vi "Perform measurements.vi"(6 "measurement configuration":T3={"Input channel"=0, "Full scale range"=10.0, "Analog source resource name"="", "Frequency"=1000.0, "Amplitude"=-1.0, "Digital capture resource name"="", "Digital capture sample rate"=800000.0, "Digital capture samples"=800000}, 11 "gRPC ID Out":T1) -> (0 "error out":errorcluster, 2 "measurement results":T2)   [LabVIEW 2021, in "AC_ADC.lvlib"]
uses:
  AC_ADC.lvlib
  Measurement Configuration.ctl
  Measurement Results.ctl
  <vilib>/gRPC/LabVIEW gRPC Library/Shared/grpcId.ctl
  shared/digitalInterface/client/dcvmDPI_AD7606B_clientImpl/dcvmDPI_AD7606B_clientImpl.lvlib
  <vilib>/gRPC/LabVIEW gRPC Library/grpc-lvsupport-release.lvlib
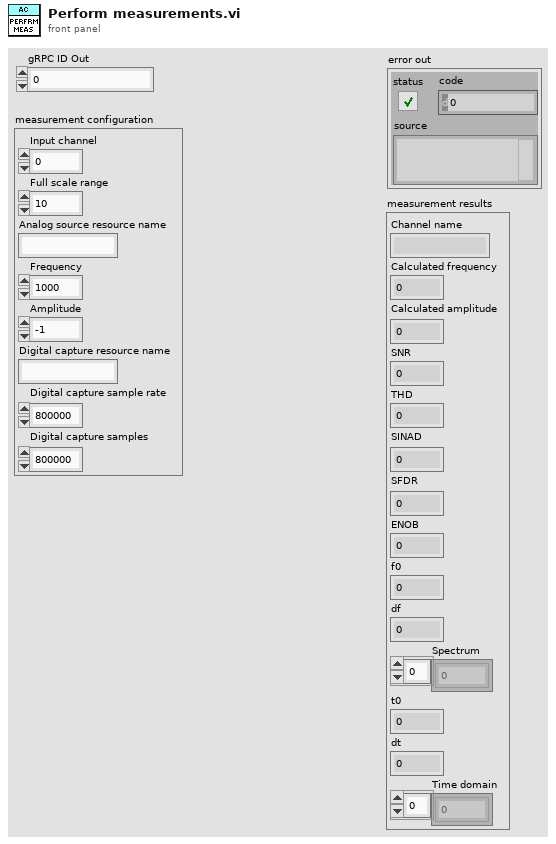
[diagram p1: front panel]
types:
  T1 = typedef "grpc-lvsupport-release.lvlib/grpcId.ctl" = u64
  T2 = typedef "AC_ADC.lvlib/Measurement Results.ctl" = cluster{"Channel name":string, "Calculated frequency":dbl, "Calculated amplitude":dbl, "SNR":dbl, "THD":dbl, "SINAD":dbl, "SFDR":dbl, "ENOB":dbl, "f0":dbl, "df":dbl, "Spectrum":dbl[], "t0":dbl, "dt":dbl, "Time domain":dbl[]}
  T3 = typedef "AC_ADC.lvlib/Measurement Configuration.ctl" = cluster{"Input channel":i32, "Full scale range":dbl, "Analog source resource name":string, "Frequency":dbl, "Amplitude":dbl, "Digital capture resource name":string, "Digital capture sample rate":dbl, "Digital capture samples":u32}
  T4 = cluster{"Detected frequency":dbl, "Detected amplitude":dbl, "SNR":dbl, "THD":dbl, "SINAD":dbl, "SFDR":dbl, "ENOB":dbl}
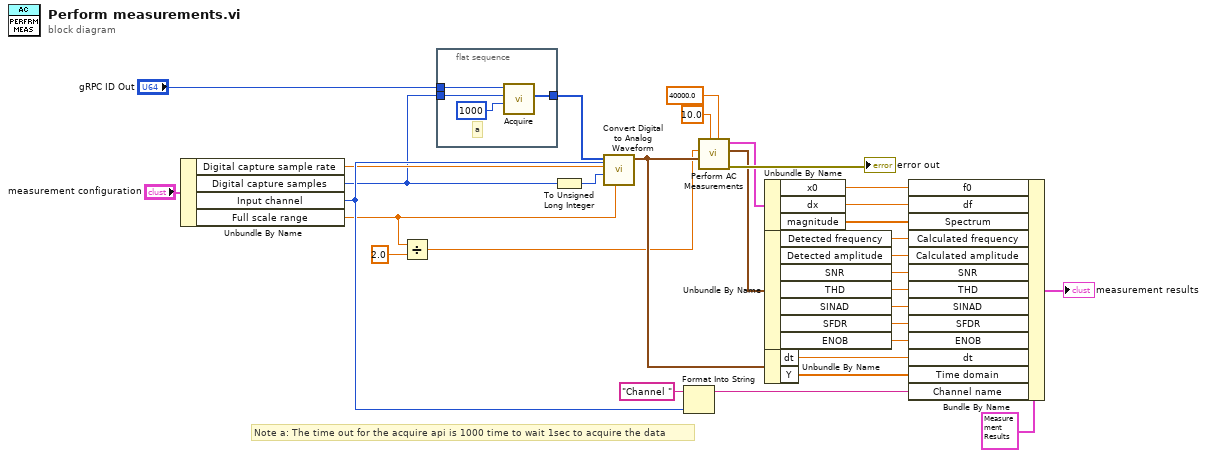
[diagram p0: block diagram]
diagram:
  # "Note a: The time out for the acquire api is 1000 time to wait 1sec to acquire the data"
  n1 = Unbundle By Name("measurement configuration") -> ("Digital capture sample rate"=w7:dbl, "Digital capture samples"=w1:u32, "Input channel"=w10:i32, "Full scale range"=w4:dbl)
  n2 = Divide(x=w4, y=2.0) -> (x/y=w5:dbl)
  n3 = flat-sequence {
    tunnel: "gRPC ID Out" -> [w36]
    tunnel: [w35] -> w2
    tunnel: w1 -> [w34]
    frame #0 {
      # "a"
      n4 = call "Acquire.vi"("Timeout (ms)"=1000, "Digital capture samples"=w34, "gRPC session in"=w36) -> ("Digital waveform"=w35:u32[])  [unwired: 6 in, 2 out]
    }
  }
  n5 = To Unsigned Long Integer(number=w1) -> (unsigned 32bit integer=w31:u32)
  n6 = call "Convert Digital to Analog Waveform.vi"("full scale range"=w4, "channel index"=w10, "Number of samples"=w31, "Sample rate"=w7, "Digital waveform in"=w2) -> ("Waveform"=w14:waveform(dbl))  [unwired: 4 in, 2 out]
  n7 = Format Into String(initial string="Channel ", w10) -> (resulting string=w8:string)  [unwired: 2 in, 1 out]
  n8 = call "Perform AC Measurements.vi"("stop frequency"=40000.0, "start frequency"=10.0, "analog waveform"=w14, "input range (pk)"=w5) -> ("error out"=→"error out":errorcluster, "AC measurement results"=w22:T4, "frequency domain"=w26:cluster{"x0":dbl, "dx":dbl, "magnitude":dbl[]})  [unwired: 5 in]
  n9 = Unbundle By Name(w26) -> ("x0"=w25:dbl, "dx"=w24:dbl, "magnitude"=w23:dbl[])
  n10 = Unbundle By Name(w22) -> ("Detected frequency"=w21:dbl, "Detected amplitude"=w20:dbl, "SNR"=w19:dbl, "THD"=w18:dbl, "SINAD"=w17:dbl, "SFDR"=w16:dbl, "ENOB"=w15:dbl)
  n11 = Unbundle By Name(w14) -> ("dt"=w13:dbl, "Y"=w12:dbl[])
  n12 = Bundle By Name(cluster=T2 {"Channel name"="", "Calculated frequency"=0.0, "Calculated amplitude"=0.0, "SNR"=0.0, "THD"=0.0, "SINAD"=0.0, "SFDR"=0.0, "ENOB"=0.0, "f0"=0.0, "df"=0.0, "Spectrum"=[], "t0"=0.0, "dt"=0.0, "Time domain"=[]} ("Measurement Results"), "f0"=w25, "df"=w24, "Spectrum"=w23, "Calculated frequency"=w21, "Calculated amplitude"=w20, "SNR"=w19, "THD"=w18, "SINAD"=w17, "SFDR"=w16, "ENOB"=w15, "dt"=w13, "Time domain"=w12, "Channel name"=w8) -> (→"measurement results":T2)
